vi "svx_Two Axis Accelerometer (simulated).vi"(6 "sampling info":cluster{"Fs":dbl, "#s":dbl}={"Fs"=51200.0, "#s"=8192.0} {"#s" format="%.2p"; "Fs" format="%.2p"}, 7 "noise amplitude":dbl=0.01 format="%.2f", 8 "error in (no error)":errorcluster, 10 "Y Axis Accelerometer":T1={"fundamental"=25.0, "Amplitude"=1.0, "phase"=90.0, "harmonics"=enum."odd only", "# of harmonics"=8} {"phase" format="%.2f"; "Amplitude" format="%.2f"; "fundamental" format="%.2f"}, 11 "X Axis Accelerometer":T1={"fundamental"=25.0, "Amplitude"=1.0, "phase"=0.0, "harmonics"=enum."odd only", "# of harmonics"=4} {"phase" format="%.2f"; "Amplitude" format="%.2f"; "fundamental" format="%.2f"}) -> (0 "error out":errorcluster, 3 "Acceleration Signals":waveform(dbl)[](graph)=[{"t0"=timestamp(0 s since 1904-01-01), "dt"=1.953125e-05, "Y"=array[8192 elements]}, {"t0"=timestamp(0 s since 1904-01-01), "dt"=1.953125e-05, "Y"=array[8192 elements]}])   [LabVIEW 2017]
doc: "Simulates two channels of dynamic data that contain a fundamental component and some harmonic content."
uses:
  <vilib>/addons/_NISVFA/_Shared subVIs/Controls/svc_Channel Info.ctl
  <vilib>/addons/_NISVFA/_Shared subVIs/Controls/svc_Engineering Units Text Ring.ctl
  <vilib>/addons/_NISVFA/_Shared subVIs/Controls/svc_Weighting Filter Text Ring.ctl
  <vilib>/addons/Sound and Vibration/svt_Calibration/SVL Scale Voltage to EU (N Ch - 1 Info).vi
  <vilib>/addons/Sound and Vibration/svt_Calibration/SVL Scale Voltage to EU (1 Ch).vi
  <vilib>/addons/_NISVFA/_Shared subVIs/Common/svc_Set SV Channel Info.vi
  <vilib>/addons/_NISVFA/_Shared subVIs/Common/svc_Set SV Channel Info (variant).vi
  <vilib>/addons/_NISVFA/_Shared subVIs/Common/SVL Set dB Reference (variant).vi
  <vilib>/addons/_NISVFA/_Shared subVIs/Common/svc_Caller VI Returned in Error Source.vi
  <vilib>/addons/_NISVFA/_Shared subVIs/Common/svc_Engineering Units to Unit Label.vi
  <vilib>/addons/_NISVFA/_Shared subVIs/Common/svc_Set dB ref if Pascal.vi
  <vilib>/addons/_NISVFA/_Shared subVIs/Common/svc_Compute Scale Factor to Convert C to EU.vi
  <vilib>/addons/_NISVFA/_Shared subVIs/Common/svc_Compute Scale Factor to Convert V to EU.vi
  <vilib>/addons/Sound and Vibration/svt_Calibration/SoundVib_Calibration.lvlib
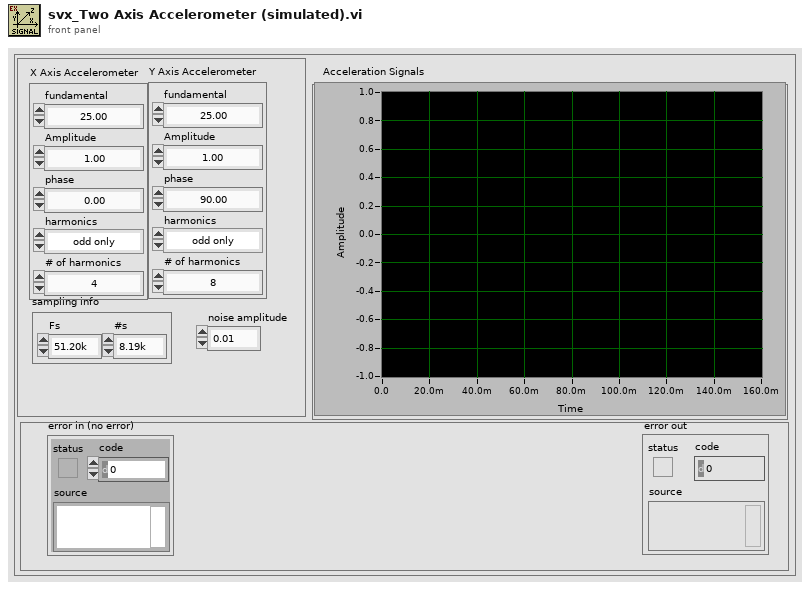
[diagram p1: front panel]
types:
  T1 = cluster{"fundamental":dbl, "Amplitude":dbl, "phase":dbl, "harmonics":enum16{"All", "odd only", "even only", "Custom frequencies"}, "# of harmonics":i32}
  T2 = typedef "svc_Channel Info.ctl" = cluster{"sensor sensitivity":dbl, "engineering units":T3, "dB reference":dbl, "custom label":string, "weighting filter":T4, "pregain":dbl}
  T3 = typedef "svc_Engineering Units Text Ring.ctl" = u16
  T4 = typedef "svc_Weighting Filter Text Ring.ctl" = u16
  T5 = enum16{"All", "odd only", "even only", "Custom frequencies"}
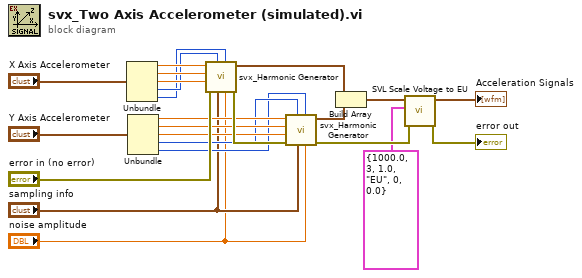
[diagram p0: block diagram]
diagram:
  n1 = Unbundle("X Axis Accelerometer") -> ("fundamental"=w18:dbl, "Amplitude"=w17:dbl, "phase"=w16:dbl, "harmonics"=w15:T5, "# of harmonics"=w14:i32)
  n2 = Unbundle("Y Axis Accelerometer") -> ("fundamental"=w13:dbl, "Amplitude"=w12:dbl, "phase"=w11:dbl, "harmonics"=w10:T5, "# of harmonics"=w9:i32)
  n3 = call <vilib>:"svx_Harmonic Generator.vi"("noise amplitude"="noise amplitude", "# of harmonics"=w14, "sampling info"="sampling info", "harmonics"=w15, "error in (no error)"="error in (no error)", "phase"=w16, "Amplitude"=w17, "fundamental"=w18) -> ("error out"=w19:errorcluster, "Waveform"=w7:waveform(dbl))  [unwired: 2 in]
  n4 = call <vilib>:"svx_Harmonic Generator.vi"("noise amplitude"="noise amplitude", "# of harmonics"=w9, "sampling info"="sampling info", "harmonics"=w10, "error in (no error)"=w19, "phase"=w11, "Amplitude"=w12, "fundamental"=w13) -> ("error out"=w3:errorcluster, "Waveform"=w20:waveform(dbl))  [unwired: 2 in]
  n5 = Build Array(w7, w20) -> (w5:waveform(dbl)[])
  n6 = call-poly <vilib>:"SVL Scale Voltage to EU.vi"("error in (no error)"=w3, "channel info"=T2 {"sensor sensitivity"=1000.0, "engineering units"=3, "dB reference"=1.0, "custom label"="EU", "weighting filter"=0, "pregain"=0.0}, "signals [V]"=w5) -> ("error out"=→"error out":errorcluster, "scaled signals [EU]"=→"Acceleration Signals":waveform(dbl)[])  [unwired: 6 in, 1 out]
